vi "Get StaticVIReference from Terminal.vi"(11 "SubVI in":refnum<vi>) -> (3 "String":string)   [LabVIEW 2014]
doc: "Traverse wire specified by connected terminal and returns StaticvVIReference object connected to other end of wire."
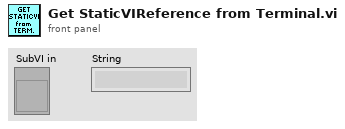
[diagram p1: front panel]
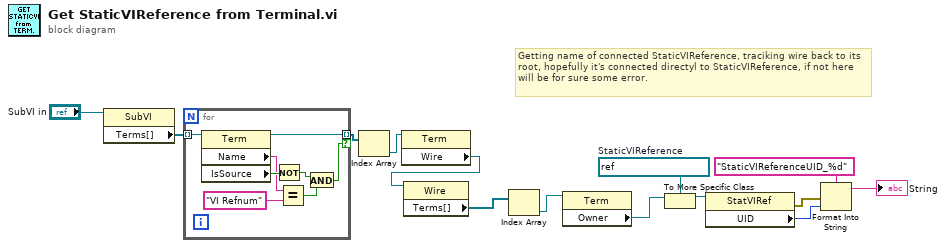
[diagram p0: block diagram]
diagram:
  w9 = refnum<vi> refnum  # StaticVIReference
  # "Getting name of connected StaticVIReference, traciking wire back to its root, hopefully it's connected directyl to StaticVIReference, if not here will be for sure some error."
  n1 = property class="SubVI"(reference="SubVI in") -> ("Terms[]"=w2:refnum<vi>[])  [unwired: 1 in, 2 out]
  n2 = for {
    tunnel: w2 -> [w22] mode=indexing
    tunnel: [w20] -> w3 mode=indexing if=w15
    n3 = property class="Term"(reference=w22) -> (reference out=w20:refnum<vi>, "Name"=w19:string, "IsSource"=w21:bool)  [unwired: 1 in, 1 out]
    n4 = Not(x=w21) -> (.not. x?=w17:bool)
    n5 = Equal?(x=w19, y="VI Refnum") -> (x = y?=w16:bool)
    n6 = And(x=w17, y=w16) -> (x .and. y?=w15:bool)
  }
  n7 = Index Array(array=w3) -> (element=w4:refnum<vi>)  [unwired: 1 in]
  n8 = property class="Term"(reference=w4) -> ("Wire"=w5:refnum<vi>)  [unwired: 1 in, 2 out]
  n9 = property class="Wire"(reference=w5) -> ("Terms[]"=w6:refnum<vi>[])  [unwired: 1 in, 2 out]
  n10 = Index Array(array=w6) -> (element=w7:refnum<vi>)  [unwired: 1 in]
  n11 = property class="Term"(reference=w7) -> ("Owner"=w8:refnum<vi>)  [unwired: 1 in, 2 out]
  n12 = To More Specific Class(target class=w9, reference=w8) -> (specific class reference=w10:refnum<vi>)  [unwired: 1 in, 1 out]
  n13 = property class="StatVIRef"(reference=w10) -> (error out=w11:errorcluster, "UID"=w14:i32)  [unwired: 1 in, 1 out]
  n14 = Format Into String(format string="StaticVIReferenceUID_%d", error in=w11, w14) -> (resulting string=→"String":string)  [unwired: 1 in, 1 out]
